vi "peakFinding getLimitIdx.vi"(8 "error in (no error)":errorcluster, 10 "peakIdxArray":i32[](array[numeric]), 11 "1stDiffData":dbl[](array[numeric])) -> (0 "error out":errorcluster, 2 "rightIdx":i32[](array[numeric]), 3 "leftIdx":i32[](array[numeric]))   [LabVIEW 2018]
uses:
  <vilib>/ptbypt/NI_PtbyPt.lvlib
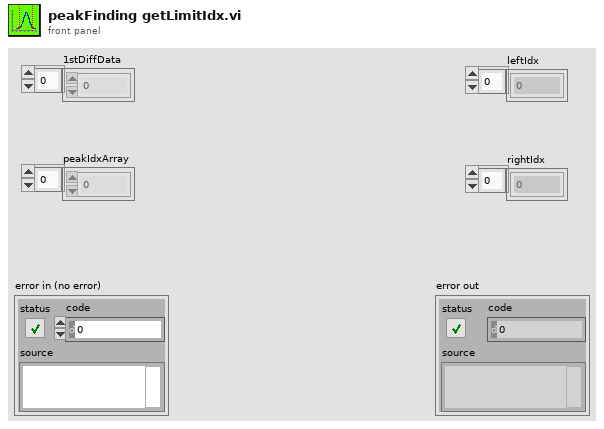
[diagram p1: front panel]
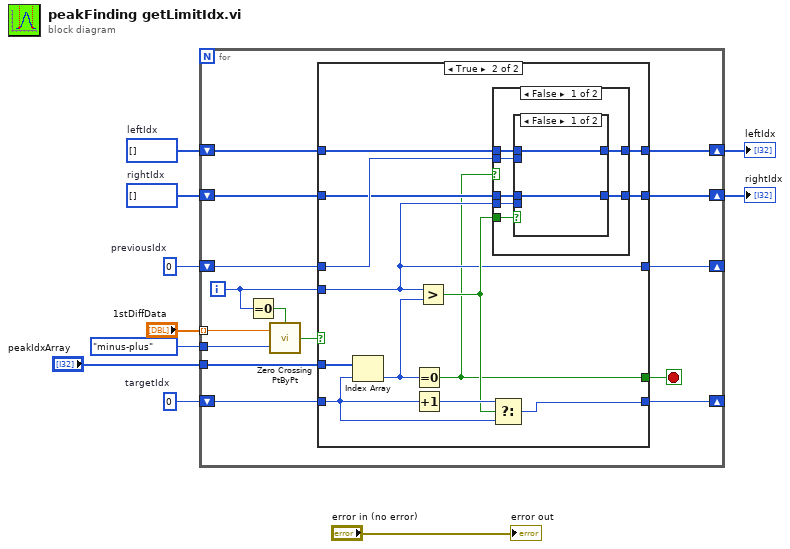
[diagram p0: block diagram]
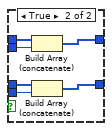
[diagram p3: hidden frame]
diagram:
  w4 = 0  # targetIdx
  w8 = 0  # previousIdx
  w9 = i32[] []  # rightIdx
  w10 = i32[] []  # leftIdx
  n1 = for {
    tunnel: "1stDiffData" -> [w25] mode=indexing
    tunnel: enum16{"either", "minus-plus", "plus-minus"}."minus-plus" ("direction") -> [w24]
    tunnel: "peakIdxArray" -> [w20]
    shift-right: [w18] -> _
    shift-left: w4 -> [w19]
    shift-right: [w17] -> _
    shift-left: w8 -> [w16]
    shift-right: [w12] -> w3
    shift-left: w10 -> [w14]
    shift-right: [w13] -> w2
    shift-left: w9 -> [w15]
    i -> [w21]
    stop <- w11 stop-if-true
    n2 = Equal To 0?(x=w21) -> (x = 0?=w23:bool)
    n3 = call <vilib>:"Zero Crossing PtByPt.vi"("initialize"=w23, "direction"=w24, "input data point"=w25) -> ("crossing"=w22:bool)
    n4 = case shown="True" w22 {
      tunnel: w21 -> [_ w36]
      tunnel: w20 -> [_ w42]
      tunnel: w19 -> [w28 w40]
      tunnel: [w28 w39] -> w18
      tunnel: [w29 w36] -> w17
      tunnel: w16 -> [w29 w37]
      tunnel: w15 -> [w26 w35]
      tunnel: w14 -> [w27 w34]
      tunnel: [w26 w33] -> w13
      tunnel: [w27 w32] -> w12
      tunnel: [_ w30] -> w11
      frame False {
      }
      frame True {
        n5 = Index Array(array=w42, index=w40) -> (element=w31:i32)
        n6 = Equal To 0?(x=w31) -> (x = 0?=w30:bool)
        n7 = Increment(x=w40) -> (x+1=w41:i32)
        n8 = Greater?(x=w36, y=w31) -> (0:w38:bool)
        n9 = case shown="False" w30 {
          tunnel: w38 -> [w49 _]
          tunnel: w37 -> [w48 _]
          tunnel: w36 -> [w47 _]
          tunnel: w35 -> [w46 w58]
          tunnel: w34 -> [w45 w59]
          tunnel: [w44 w58] -> w33
          tunnel: [w43 w59] -> w32
          frame False {
            n10 = case shown="False" w49 {
              tunnel: w48 -> [_ w56]
              tunnel: w47 -> [_ w54]
              tunnel: w46 -> [w50 w55]
              tunnel: w45 -> [w51 w57]
              tunnel: [w50 w53] -> w44
              tunnel: [w51 w52] -> w43
              frame False {
              }
              frame True {
                n11 = Build Array (concatenate)(w57, w56) -> (w52:i32[])
                n12 = Build Array (concatenate)(w55, w54) -> (w53:i32[])
              }
            }
          }
          frame True {
          }
        }
        n13 = Select(t=w41, s=w38, f=w40) -> (s? t:f=w39:i32)
      }
    }
  }
  "leftIdx" <- w3
  "rightIdx" <- w2
  "error out" <- "error in (no error)"
